vi "Flock_Shared_LaunchProcess_WriteMessage.vi"(4 "Show Front Panel?":bool, 6 "Reentrant?":bool=TRUE, 7 "VI Path":path, 8 "error in (no error)":errorcluster, 9 "Initial Message Value":string, 10 "Initial Message Name":string, 11 "Process List":T1) -> (0 "error out":errorcluster)   [LabVIEW 2014, in "Flock_Shared_Messaging.lvlib"]
doc: "This VI asynchronously launches a specified VI with parameters. The VI must have a connector pane that contains only the Process List typedef in the top left terminal (see block diagram).\n\nThe specified VI will likely implement the AMC inspired Flock template."
uses:
  Flock_Shared_Messaging.lvlib
  LocalProcessMessaging/Flock_Shared_LocalProcessMessaging.lvlib
  ProcessList.ctl
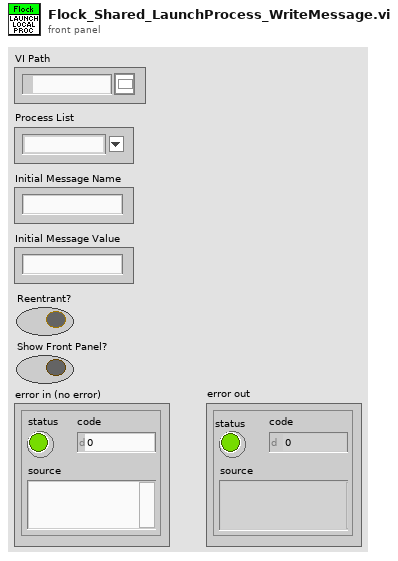
[diagram p1: front panel]
types:
  T1 = typedef "Flock_Shared_Messaging.lvlib/ProcessList.ctl" = string
  T2 = enum32{"Invalid", "Standard", "Closed", "Hidden", "Minimized", "Maximized"}
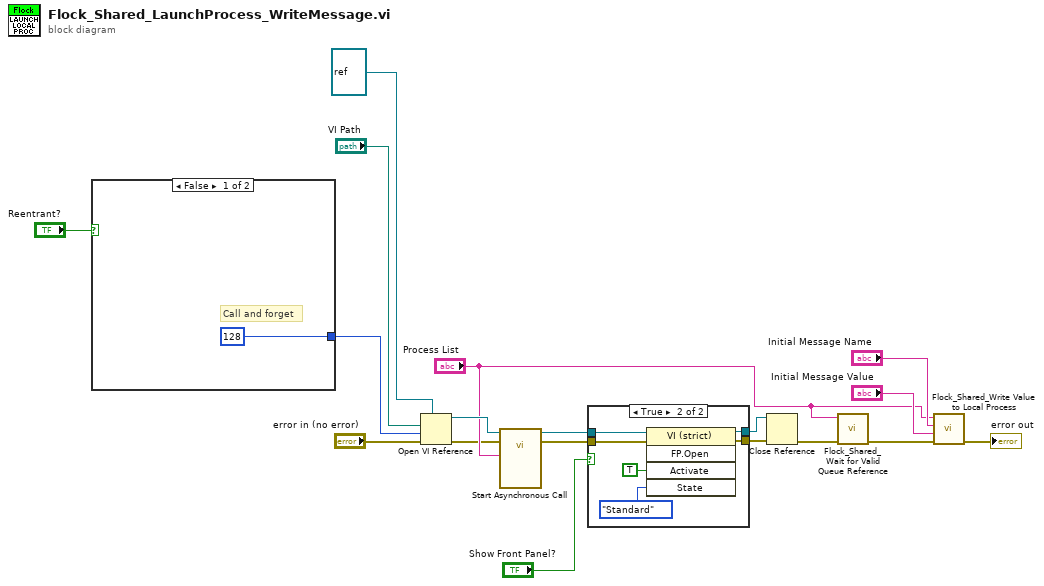
[diagram p0: block diagram]
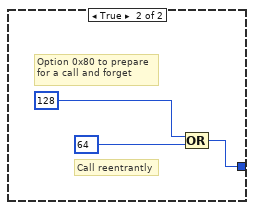
[diagram p3: hidden frame]
diagram:
  n1 = case shown="False" "Reentrant?" {
    tunnel: [128 ("options") w20] -> w18
    frame False {
      # "Call and forget"
    }
    frame True {
      # "Option 0x80 to prepare\nfor a call and forget"
      # "Call reentrantly"
      n2 = Compound Arithmetic op=OR(128 ("options"), 64 ("options")) -> (w20:i32)
    }
  }
  n3 = Open VI Reference(type specifier VI Refnum (for type only)=refnum<vi> refnum, vi path="VI Path", options=w18, error in (no error)="error in (no error)") -> (vi reference=w17:refnum<vi>, error out=w8:errorcluster)  [unwired: 2 in]
  n4 = call-by-ref "Start Asynchronous Call"(reference=w17, error in=w8, "Process List"="Process List") -> (reference out=w5:refnum<vi>, error out=w4:errorcluster)  [unwired: 11 in]
  n5 = case shown="True" "Show Front Panel?" {
    tunnel: w5 -> [w24 w30]
    tunnel: w4 -> [w23 w29]
    tunnel: [w23 w28] -> w3
    tunnel: [w24 w27] -> w2
    frame False {
    }
    frame True {
      n6 = invoke class="VI (strict)" method="FP.Open"(reference=w30, error in=w29, "Activate"=TRUE ("Activate?"), "State"=T2."Standard") -> (reference out=w27:refnum<vi>, error out=w28:errorcluster)  [unwired: 1 in, 3 out]
    }
  }
  n7 = Close Reference(reference=w2, error in (no error)=w3) -> (error out=w6:errorcluster)
  n8 = call "Flock_Shared_Wait for Valid Queue Reference.vi"("error in (no error)"=w6, "Process List"="Process List") -> ("error out"=w10:errorcluster)  [unwired: 7 in, 2 out]
  n9 = call "Flock_Shared_Write Value to Local Process.vi"("error in (no error)"=w10, "Message Value"="Initial Message Value", "Message Name"="Initial Message Name", "Process List"="Process List") -> ("error out"=→"error out":errorcluster)  [unwired: 7 in]
